vi "__RunTestsInCurrentProject.vi"() -> ()   [LabVIEW 2019]
uses:
  TestResult/TestResult.lvclass
  TestRunner/TestRunner.lvclass
  TestSuite.lvclass
  TestFailure/TestFailure.lvclass
panel:
  out "Count":i32
  out "error out":errorcluster
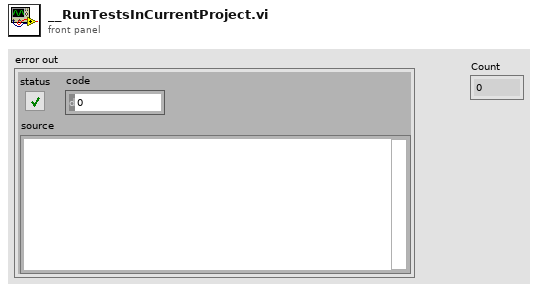
[diagram p1: front panel]
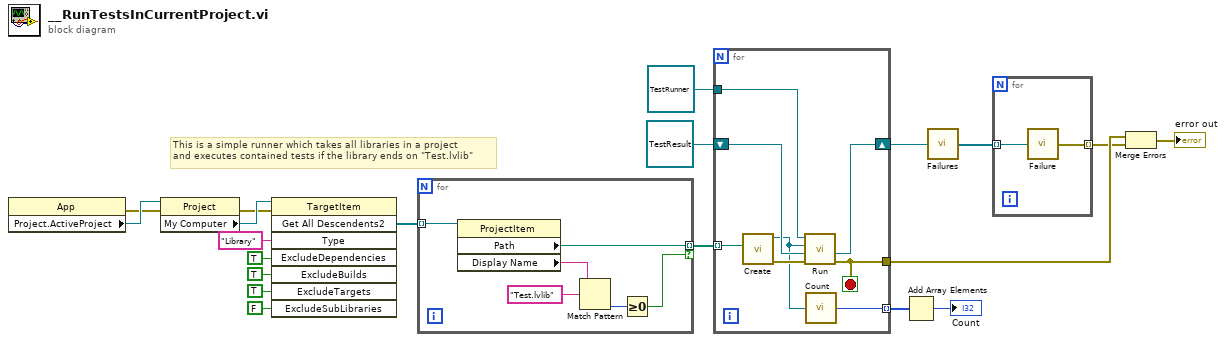
[diagram p0: block diagram]
diagram:
  # "This is a simple runner which takes all libraries in a project\nand executes contained tests if the library ends on \"Test.lvlib\""
  n1 = property class="App"() -> (error out=w18:errorcluster, "Project.ActiveProject"=w20:refnum<vi>)  [unwired: 2 in, 1 out]
  n2 = property class="Project"(reference=w20, error in=w18) -> (error out=w17:errorcluster, "My Computer"=w19:refnum<vi>)  [unwired: 1 out]
  n3 = invoke class="TargetItem" method="Get All Descendents2"(reference=w19, error in=w17, "Type"="Library", "ExcludeDependencies"=TRUE, "ExcludeBuilds"=TRUE, "ExcludeTargets"=TRUE, "ExcludeSubLibraries"=FALSE) -> ("Get All Descendents2"=w11:refnum<vi>[])  [unwired: 1 in, 7 out]
  n4 = for {
    tunnel: w11 -> [w26] mode=indexing
    tunnel: [w22] -> w10 mode=indexing if=w21
    n5 = property class="ProjectItem"(reference=w26) -> ("Path"=w22:path, "Display Name"=w23:string)  [unwired: 1 in, 2 out]
    n6 = Match Pattern(string=w23, regular expression="Test.lvlib") -> (offset past match=w24:i32)  [unwired: 1 in, 3 out]
    n7 = Greater Or Equal To 0?(x=w24) -> (x >= 0?=w21:bool)
  }
  n8 = for {
    tunnel: w10 -> [w34] mode=indexing
    shift-right: [w32] -> w8
    shift-left: refnum<class "TestResult.lvclass"> refnum ("TestResult out") -> [w33]
    tunnel: [w30] -> w6
    tunnel: refnum<class "TestRunner.lvclass"> refnum ("TestRunner in") -> [w29]
    tunnel: [w27] -> w2 mode=indexing
    stop <- w30 stop-if-true
    n9 = call "Create.vi"("Path"=w34) -> ("error out"=w31:errorcluster, "TestSuite"=w28:refnum<class "TestSuite.lvclass">)  [unwired: 9 in]
    n10 = call-dynamic "Run.vi"("error in (no error)"=w31, "TestResult"=w33, "TestSuite"=w28, "TestRunner in"=w29) -> ("error out"=w30:errorcluster, "TestResult out"=w32:refnum<class "TestResult.lvclass">)  [unwired: 5 in, 1 out]
    n11 = call "Count.vi"("TestSuite In"=w28) -> ("Count"=w27:i32)
  }
  n12 = Add Array Elements(numeric array=w2) -> (sum=→"Count":i32)
  n13 = call "Failures.vi"("TestResult In"=w8) -> ("Failures"=w7:refnum<class "TestFailure.lvclass">[])
  n14 = for {
    tunnel: w7 -> [w36] mode=indexing
    tunnel: [w35] -> w5 mode=indexing
    n15 = call "Failure.vi"("TestFailure In"=w36) -> ("Failure"=w35:errorcluster)
  }
  n16 = Merge Errors(w6, w5) -> (→"error out":errorcluster)
